vi "GPS -Markers Add to Collection.vi"(0 ".NET Refnum in":refnum<k24>, 1 "Inputs":T2) -> (8 "arrOverlayRefs":refnum<k24>[](array[refnum]), 12 ".NET Refnum in":refnum<k24>, 14 "RefPointsColl -OUT":refnum<k24>, 15 "arrPtKyOrId":string[](array[string]), 16 "arrLat|LngActv":dbl[][](array[numeric]), 17 "MarkersCount":i32, 18 "QFNs":cluster{"FN":T3, "Data":variant}[](array[cluster]))   [LabVIEW 2019]
uses:
  \\mac\Dropbox/gmap.net/GMAP.NET 8.6/data/GMap.NET.WindowsForms.dll
  data/GMap.NET.WindowsForms.dll
  ctlSeqFNs -GPSLocation.ctl
  ctlInput4PtsColl.ctl
  \\mac\Dropbox/gmap.net/GMAP.NET 8.6/data/GMap.NET.Core.dll
  data/GMap.NET.Core.dll
  System.Drawing
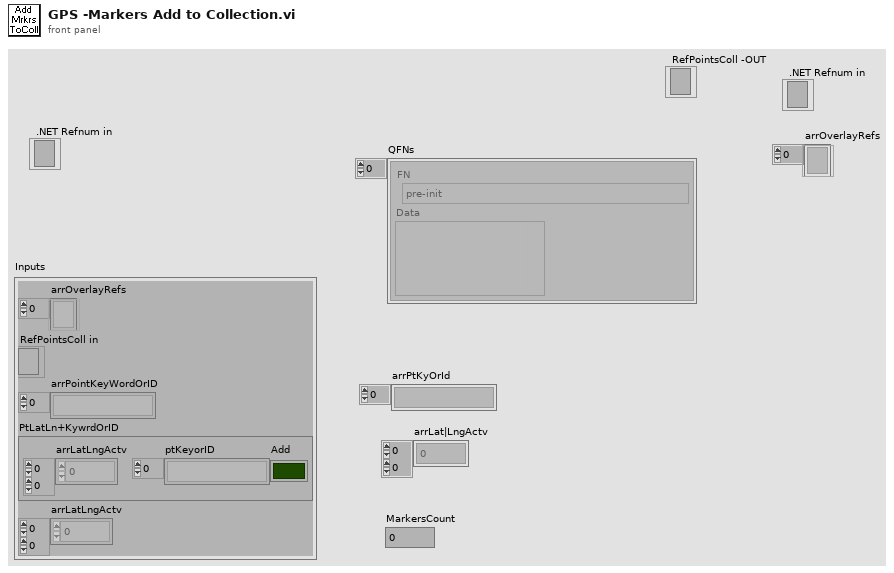
[diagram p1: front panel]
types:
  T1 = typedef "ctlInput4PtsColl.ctl" = cluster{"arrLatLngActv":dbl[][], "ptKeyorID":string[], "Add":bool}
  T2 = cluster{"arrOverlayRefs":refnum<k24>[], "RefPointsColl in":refnum<k24>, "arrPointKeyWordOrID":string[], "PtLatLn+KywrdOrID":T1, "arrLatLngActv":dbl[][]}
  T3 = typedef "ctlSeqFNs -GPSLocation.ctl" = enum16{"pre-init", "preinit01", "preinit02", "preinit03", "preinit04", "preinit05", "init", "idle", "GUI -Pop Menu", "GUI -Add Marker Combo", "GUI -Annotate Grid", "ALIGN COLS", "SET -Provider", "SET -SCALE", "OVERLAY -ADD", "POINTS -CREATE LIST (Container)", "MARKERS -CREATE LIST", "MAP -MARKER Add Or Rmv", "DOWNLOAD -Project Addr", "MAP -Marker Update", "MAP -Save", "MAP -Markers Autofit", "MAP -Addr to Lat + Lng", "MAP -Markers Clear", "PIN DROP -Get Nearest", "AUDIT -Use Marker Shown", "error", "exit"}
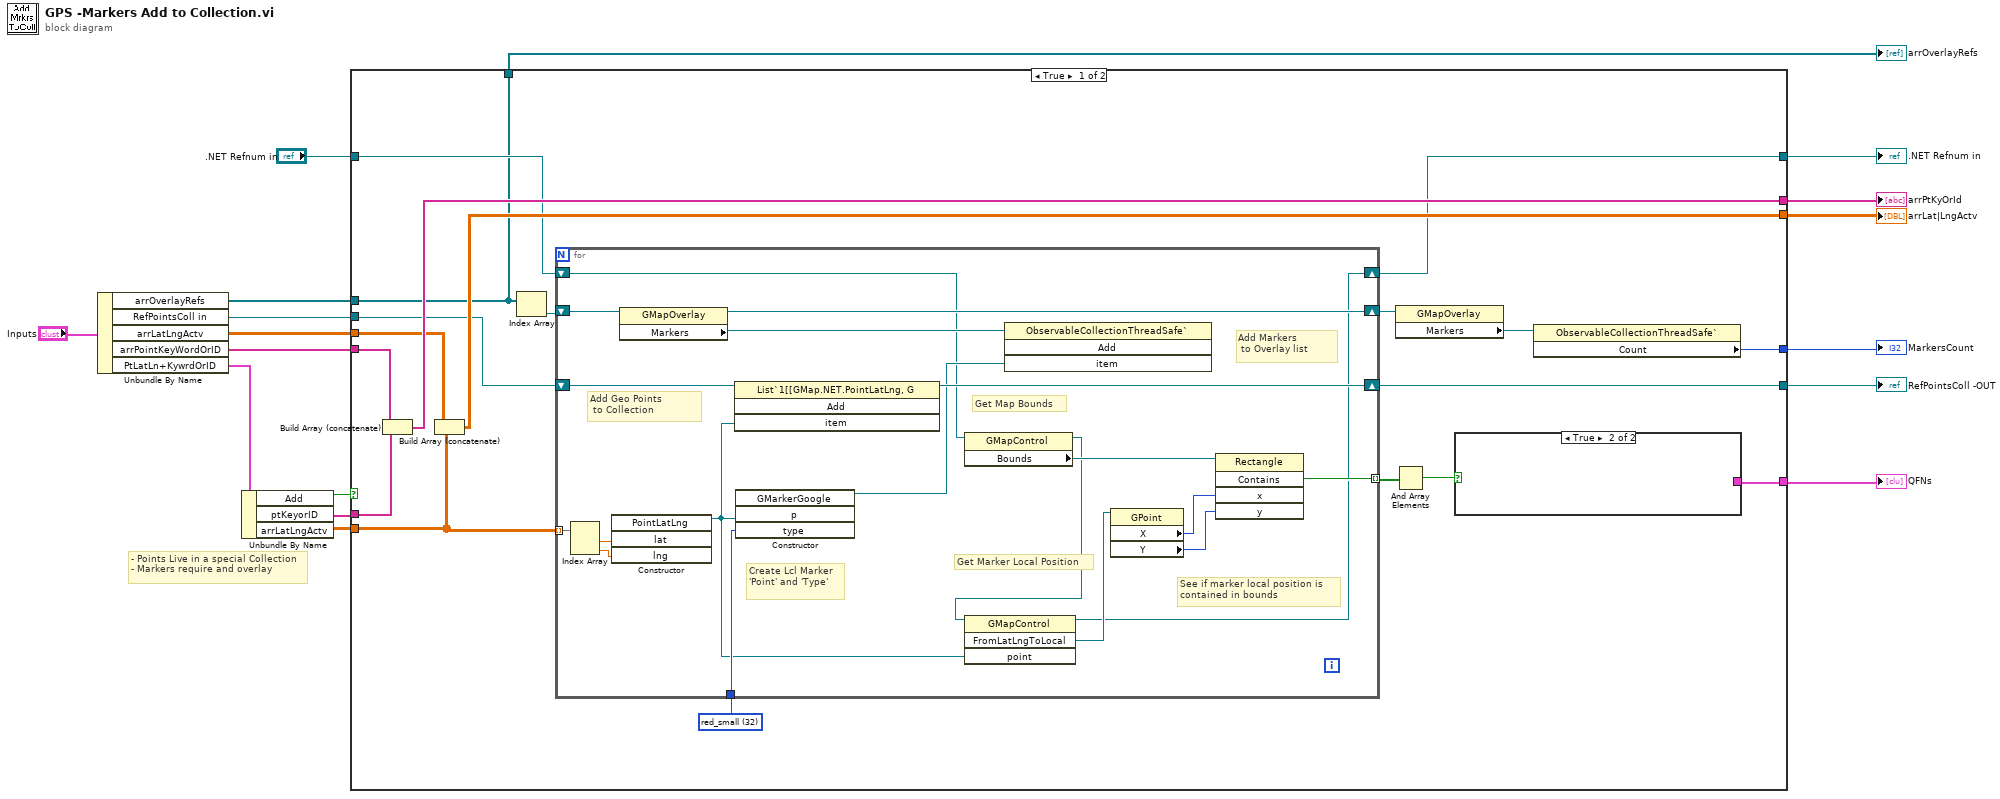
[diagram p0: block diagram]
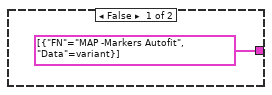
[diagram p2: hidden frame]
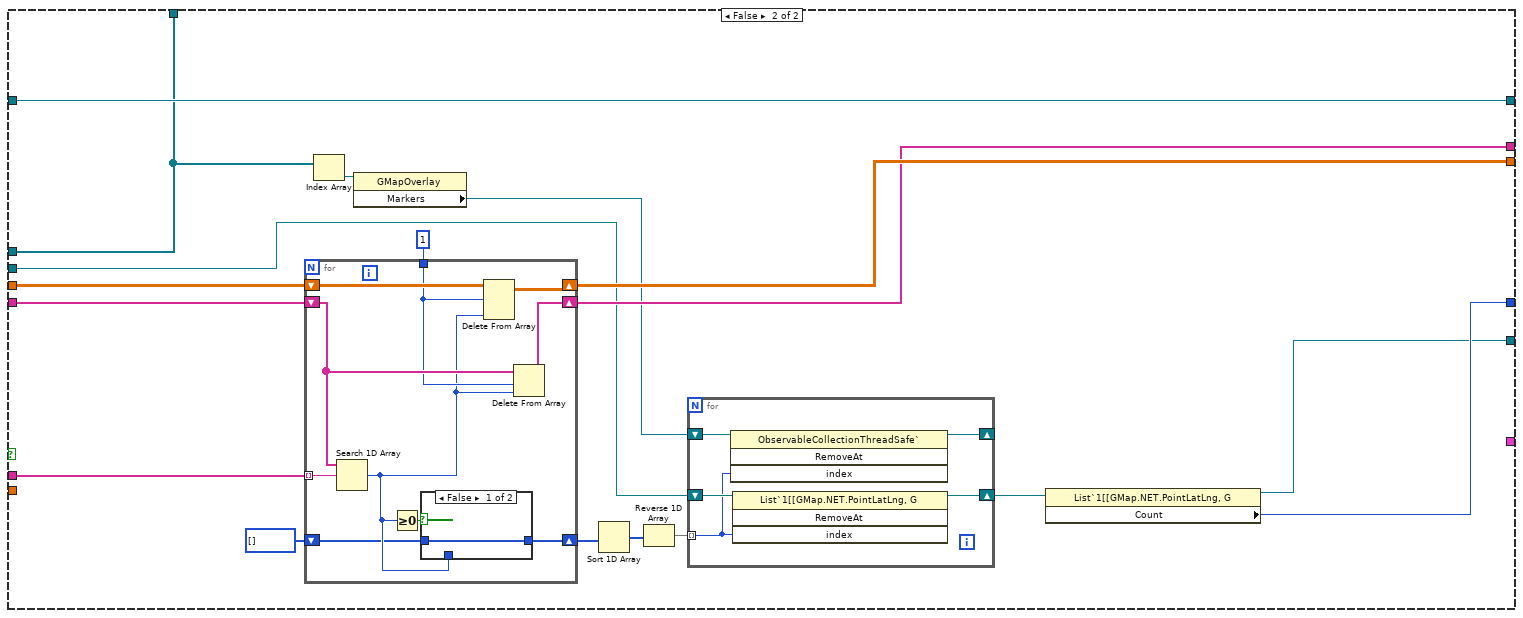
[diagram p3: hidden frame]
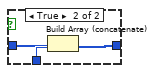
[diagram p4: hidden frame]
diagram:
  # "- Points Live in a special Collection\n- Markers require and overlay"
  n1 = Unbundle By Name("Inputs") -> ("arrOverlayRefs"=w9:refnum<k24>[], "RefPointsColl in"=w8:refnum<k24>, "arrLatLngActv"=w7:dbl[][], "arrPointKeyWordOrID"=w5:string[], "PtLatLn+KywrdOrID"=w6:T1)
  n2 = Unbundle By Name(w6) -> ("Add"=w1:bool, "ptKeyorID"=w11:string[], "arrLatLngActv"=w12:dbl[][])
  n3 = case shown="True" w1 {
    tunnel: [w36 _] -> w17
    tunnel: [w35 w68] -> w16
    tunnel: [w30 w69] -> w15
    tunnel: [w29 w70] -> w14
    tunnel: [w28 w59] -> w13
    tunnel: w12 -> [w27 _]
    tunnel: w11 -> [w26 w73]
    tunnel: w9 -> [w19 w57]
    tunnel: w8 -> [w25 w61]
    tunnel: w7 -> [w24 w72]
    tunnel: w5 -> [w23 w74]
    tunnel: ".NET Refnum in" -> [w20 w58]
    tunnel: [w18 w58] -> w2
    tunnel: [w19 w57] -> w3
    frame True {
      w32 = 32 items=["none", "arrow", "blue", "blue_small", "blue_dot", "blue_pushpin", "brown_small", "gray_small", "green", "green_small", "green_dot", "green_pushpin", "green_big_go", "yellow", "yellow_small", "yellow_dot", "yellow_big_pause", "yellow_pushpin", "lightblue", "lightblue_dot", "lightblue_pushpin", "orange", "orange_small", "orange_dot", "pink", "pink_dot", "pink_pushpin", "purple", "purple_small", "purple_dot", "purple_pushpin", "red", "red_small", "red_dot", "red_pushpin", "red_big_stop", "black_small", "white_small"] ("type")
      n4 = Build Array (concatenate)(w23, w26) -> (w30:string[])
      n5 = Build Array (concatenate)(w24, w27) -> (w29:dbl[][])
      n6 = Index Array(array=w19) -> (element=w31:refnum<k24>)  [unwired: 1 in]
      n7 = for {
        shift-right: [w55] -> w28
        shift-left: w25 -> [w56]
        tunnel: w27 -> [w52] mode=indexing
        shift-right: [w50] -> w33
        shift-left: w31 -> [w51]
        tunnel: w32 -> [w48]
        tunnel: [w46] -> w22 mode=indexing
        shift-right: [w38] -> w18
        shift-left: w20 -> [w44]
        # "See if marker local position is \ncontained in bounds"
        # "Get Marker Local Position"
        # "Get Map Bounds"
        # "Add Markers\n to Overlay list"
        # "Create Lcl Marker  'Point' and 'Type'"
        # "Add Geo Points\n to Collection"
        n8 = Index Array(array=w52) -> (element #1=w54:dbl, element #2=w53:dbl)  [unwired: 2 in]
        n9 = constructor class="PointLatLng"("lat"=w54, "lng"=w53) -> (reference out=w43:refnum<k24>)  [unwired: 3 in, 4 out]
        n10 = property class="GMapOverlay"(reference=w51) -> (reference out=w50:refnum<k24>, "Markers"=w49:refnum<k24>)  [unwired: 1 in, 1 out]
        n11 = invoke class="List`1[[GMap.NET.PointLatLng, G" method="Add"(reference=w56, "item"=w43) -> (reference out=w55:refnum<k24>)  [unwired: 2 in, 3 out]
        n12 = constructor class="GMarkerGoogle"("p"=w43, "type"=w48) -> (reference out=w45:refnum<k24>)  [unwired: 3 in, 4 out]
        n13 = property class="GMapControl"(reference=w44) -> (reference out=w39:refnum<k24>, "Bounds"=w47:refnum<k24>)  [unwired: 1 in, 1 out]
        n14 = invoke class="GMapControl" method="FromLatLngToLocal"(reference=w39, "point"=w43) -> (reference out=w38:refnum<k24>, "FromLatLngToLocal"=w42:refnum<k24>)  [unwired: 2 in, 2 out]
        n15 = invoke class="ObservableCollectionThreadSafe`" method="Add"(reference=w49, "item"=w45) -> ()  [unwired: 2 in, 4 out]
        n16 = property class="GPoint"(reference=w42) -> ("X"=w41:i64, "Y"=w40:i64)  [unwired: 1 in, 2 out]
        n17 = invoke class="Rectangle" method="Contains"(reference=w47, "x"=w41, "y"=w40) -> ("Contains"=w46:bool)  [unwired: 2 in, 4 out]
      }
      n18 = property class="GMapOverlay"(reference=w33) -> ("Markers"=w34:refnum<k24>)  [unwired: 1 in, 2 out]
      n19 = And Array Elements(Boolean array=w22) -> (logical AND=w21:bool)
      n20 = case shown="True" w21 {
        tunnel: [cluster{"FN":T3, "Data":variant}[] [{"FN"=enum."MAP -Markers Autofit", "Data"=variant}] ("QFNs") _] -> w36
        frame False {
        }
        frame True {
        }
      }
      n21 = property class="ObservableCollectionThreadSafe`"(reference=w34) -> ("Count"=w35:i32)  [unwired: 1 in, 2 out]
    }
    frame False {
      n22 = for {
        shift-right: [w85] -> w69
        shift-left: w74 -> [w87]
        tunnel: w73 -> [w89] mode=indexing
        shift-right: [w84] -> w70
        shift-left: w72 -> [w88]
        tunnel: 1 -> [w86]
        shift-right: [w81] -> w65
        shift-left: i32[] [] -> [w80]
        n23 = Search 1D Array(1D array=w87, element=w89) -> (index of element=w82:i32)  [unwired: 1 in]
        n24 = Greater Or Equal To 0?(x=w82) -> (x >= 0?=w83:bool)
        n25 = case shown="False" w83 {
          tunnel: w82 -> [_ w93]
          tunnel: [w90 w92] -> w81
          tunnel: w80 -> [w90 w91]
          frame False {
          }
          frame True {
            n26 = Build Array (concatenate)(w91, w93) -> (w92:i32[])
          }
        }
        n27 = Delete From Array(array=w88, length=w86, index (col)=w82) -> (array with subset deleted=w84:dbl[][])  [unwired: 1 in, 1 out]
        n28 = Delete From Array(array=w87, length=w86, index=w82) -> (array with subset deleted=w85:string[])  [unwired: 1 out]
      }
      n29 = Index Array(array=w57) -> (element=w67:refnum<k24>)  [unwired: 1 in]
      n30 = property class="GMapOverlay"(reference=w67) -> ("Markers"=w62:refnum<k24>)  [unwired: 1 in, 2 out]
      n31 = Sort 1D Array(array=w65) -> (sorted array=w64:i32[])
      n32 = Reverse 1D Array(array=w64) -> (reversed array=w63:i32[])
      n33 = for {
        shift-right: [w78] -> w60
        shift-left: w61 -> [w79]
        shift-right: [w76] -> _
        shift-left: w62 -> [w77]
        tunnel: w63 -> [w75] mode=indexing
        n34 = invoke class="ObservableCollectionThreadSafe`" method="RemoveAt"(reference=w77, "index"=w75) -> (reference out=w76:refnum<k24>)  [unwired: 2 in, 3 out]
        n35 = invoke class="List`1[[GMap.NET.PointLatLng, G" method="RemoveAt"(reference=w79, "index"=w75) -> (reference out=w78:refnum<k24>)  [unwired: 2 in, 3 out]
      }
      n36 = property class="List`1[[GMap.NET.PointLatLng, G"(reference=w60) -> (reference out=w59:refnum<k24>, "Count"=w68:i32)  [unwired: 1 in, 1 out]
    }
  }
  "QFNs" <- w17
  "MarkersCount" <- w16
  "arrPtKyOrId" <- w15
  "arrLat|LngActv" <- w14
  "RefPointsColl -OUT" <- w13
  "arrOverlayRefs" <- w3
  ".NET Refnum in" <- w2
